vi "Snap Image test.vi"(8 "error in (no error)":errorcluster, 11 "Refnum in":T2) -> (0 "error out":errorcluster, 1 "Pass ?":bool, 2 "Image Out":T1, 3 "Refnum out":T2)   [LabVIEW 2015]
uses:
  <vilib>/vision/Image Controls.llb/IMAQ Image.ctl
  <vilib>/userdefined/High Color/IMAQdx.ctl
  <vilib>/vision/driver/NI_Vision_Acquisition_Software.lvlib
panel:
  out "Process Image":T1(plugin-control)
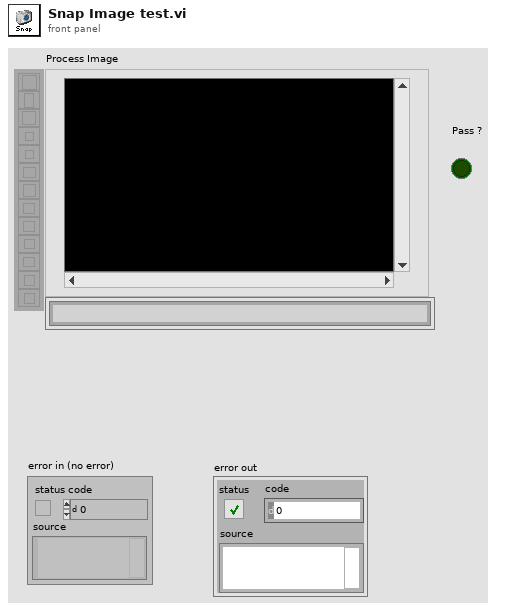
[diagram p1: front panel]
types:
  T1 = typedef "IMAQ Image.ctl" = refnum<image>
  T2 = typedef "IMAQdx.ctl" = refnum<k21>
  T3 = enum32{"Bad", "Idle", "Run top level", "Running"}
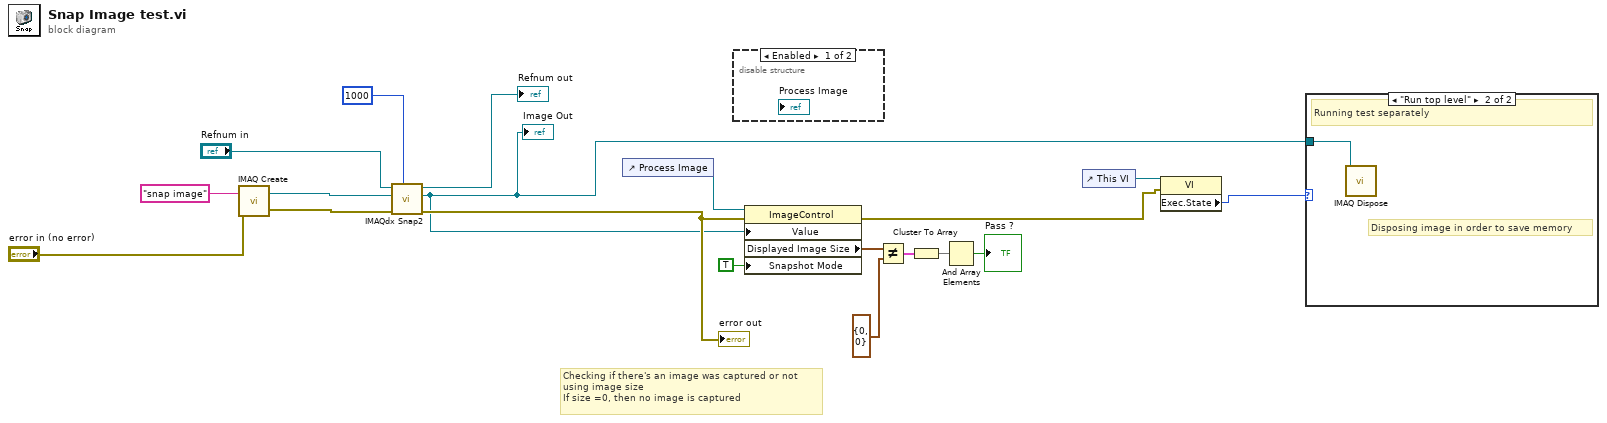
[diagram p0: block diagram]
diagram:
  # "Checking if there's an image was captured or not\nusing image size\nIf size =0, then no image is captured"
  n1 = call "IMAQ Create"("Image Name"="snap image", "error in (no error)"="error in (no error)") -> ("New Image"=w17:T1, "error out"=w19:errorcluster)  [unwired: 3 in]
  n2 = call <vilib>:"IMAQdx Snap2.vi"("Timeout (ms)"=1000, "error in"=w19, "Image In"=w17, "Session In"="Refnum in") -> ("error out"=w8:errorcluster, "Image Out"=w4:T1, "Session Out"=→"Refnum out":T2)  [unwired: 5 in]
  "error out" <- w8
  "Image Out" <- w4
  n3 = control-ref of="Process Image"() -> (w6:refnum<vi>)
  n4 = disable-structure shown="Enabled" {
    frame Enabled {
    }
    frame Disabled {
    }
  }
  n5 = property class="ImageControl"(reference=w6, error in=w8, "Value"=w4, "Snapshot Mode"=TRUE) -> (error out=w1:errorcluster, "Displayed Image Size"=w10:cluster{"Width":u32, "Height":u32})  [unwired: 1 out]
  n6 = Not Equal?(x=w10, y=cluster{"Width":u32, "Height":u32} {"Width"=0, "Height"=0} ("Displayed Image:Size:All Elements")) -> (x != y?=w12:cluster{"Width":bool, "Height":bool})
  n7 = Cluster To Array(cluster=w12) -> (array=w11:bool[])
  n8 = And Array Elements(Boolean array=w11) -> (logical AND=→"Pass ?":bool)
  n9 = control-ref of="This VI"() -> (w3:refnum<vi>)
  n10 = property class="VI"(reference=w3, error in=w1) -> ("Exec.State"=w2:T3)  [unwired: 2 out]
  n11 = case shown="\"Run top level\"" w2 {
    tunnel: w4 -> [_ w20]
    frame Default {
      # "Running within program"
    }
    frame "Run top level" {
      # "Disposing image in order to save memory"
      # "Running test separately"
      n12 = call "IMAQ Dispose"("Image"=w20) -> ()  [unwired: 5 in, 1 out]
    }
  }
